vi "ViewWindowCreate.vi"(10 "File":string="FixedHorizonTrans.png", 11 "Solid Horizon Path.PNG":path=path "C:/Users/uksayerr/Documents/My LabView/Content Creation/artificial horizon/FixedHorizonTrans.png") -> (3 "SceneObject out":refnum<vi>)   [LabVIEW 2010]
uses:
  <vilib>/picture/3D Picture Control/NI_3D Picture Control.lvlib
panel:
  # "Generates the Viewing Window with the picture \nat the path specified below"
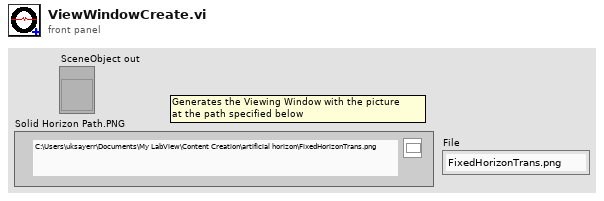
[diagram p1: front panel]
types:
  T1 = enum16{"As a Decal", "With Modulation", "With Blending", "As a replacement"}
  T2 = cluster{"Red":sgl, "Green":sgl, "Blue":sgl, "Alpha":sgl}[]
  T3 = enum16{"Overall", "Per Primitive", "Per Vertex", "Binding Off"}
  T4 = enum16{"Normal Bin", "Opaque Bin", "Transparent Bin"}
  T5 = enum16{"Points", "Lines", "Line Strip", "Line Loop", "Triangles", "Triangle Strip", "Triangle Fan", "Quads", "Quad Strip", "Polygon"}
  T6 = typedef "imagedata.ctl" = cluster{"image type":i32, "image depth":i32, "image":u8[], "mask":u8[], "colors":u32[], "Rectangle":cluster{"left":i16, "top":i16, "right":i16, "bottom":i16}}
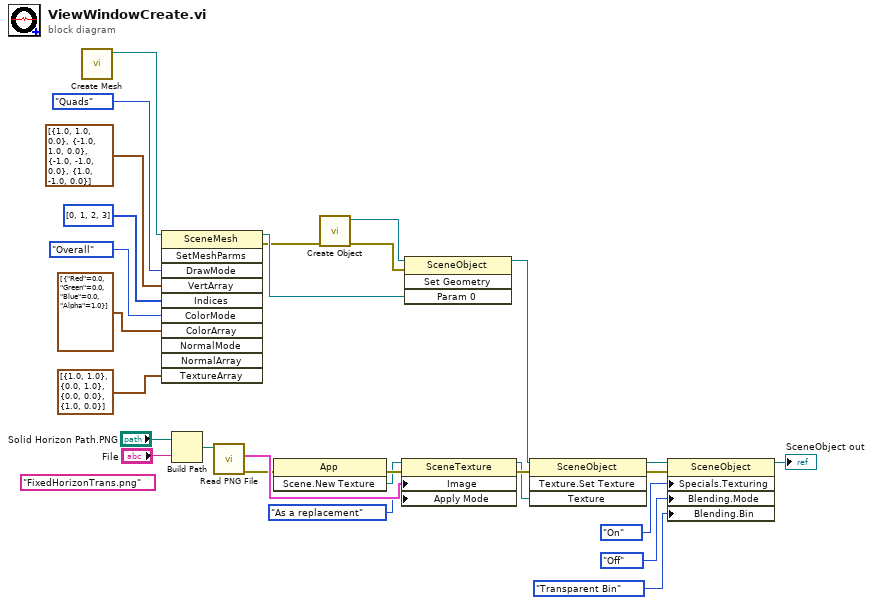
[diagram p0: block diagram]
diagram:
  (unwired) "FixedHorizonTrans.png" ("name or relative path")
  n1 = call <vilib>:"Create Mesh.vi"() -> ("New Mesh Refnum"=w12:refnum<vi>)  [unwired: 10 in, 1 out]
  n2 = invoke class="SceneMesh" method="SetMeshParms"(reference=w12, "DrawMode"=T5."Quads" ("Draw Mode"), "VertArray"=cluster{"X":sgl, "Y":sgl, "Z":sgl}[] [{"X"=1.0, "Y"=1.0, "Z"=0.0}, {"X"=-1.0, "Y"=1.0, "Z"=0.0}, {"X"=-1.0, "Y"=-1.0, "Z"=0.0}, {"X"=1.0, "Y"=-1.0, "Z"=0.0}] ("Vertex Array"), "Indices"=u32[] [0, 1, 2, 3], "ColorMode"=T3."Overall" ("Color Binding Mode"), "ColorArray"=T2 [{"Red"=0.0, "Green"=0.0, "Blue"=0.0, "Alpha"=1.0}] ("Color Array"), "TextureArray"=cluster{"S":sgl, "T":sgl}[] [{"S"=1.0, "T"=1.0}, {"S"=0.0, "T"=1.0}, {"S"=0.0, "T"=0.0}, {"S"=1.0, "T"=0.0}] ("Texture Coordinate Array")) -> (reference out=w19:refnum<vi>, error out=w17:errorcluster)  [unwired: 4 in, 9 out]
  n3 = Build Path(base path="Solid Horizon Path.PNG", name or relative path="File") -> (appended path=w2:path)
  n4 = call <vilib>:"Read PNG File.vi"("path to PNG file"=w2) -> ("error out"=w10:errorcluster, "image data"=w11:T6)  [unwired: 8 in, 1 out]
  n5 = invoke class="App" method="Scene.New Texture"(error in=w10) -> (error out=w8:errorcluster, "Scene.New Texture"=w7:refnum<vi>)  [unwired: 2 in, 1 out]
  n6 = call <vilib>:"Create Object.vi"("error in (no error)"=w17) -> ("error out"=w18:errorcluster, "Scene:New Object"=w5:refnum<vi>)  [unwired: 9 in]
  n7 = property class="SceneTexture"(reference=w7, error in=w8, "Image"=w11, "Apply Mode"=T1."As a replacement") -> (reference out=w20:refnum<vi>, error out=w21:errorcluster)
  n8 = invoke class="SceneObject" method="Set Geometry"(reference=w5, error in=w18, "Param 0"=w19) -> (reference out=w6:refnum<vi>)  [unwired: 1 in, 3 out]
  n9 = invoke class="SceneObject" method="Texture.Set Texture"(reference=w6, error in=w21, "Texture"=w20) -> (reference out=w22:refnum<vi>, error out=w23:errorcluster)  [unwired: 1 in, 2 out]
  n10 = property class="SceneObject"(reference=w22, error in=w23, "Specials.Texturing"=enum16{"Inherit Value", "Off", "On"}."On" ("Specials:Texturing"), "Blending.Mode"=enum16{"Inherit Value", "Off", "On"}."Off" ("Blending:Mode 2"), "Blending.Bin"=T4."Transparent Bin" ("Blending:Bin")) -> (reference out=→"SceneObject out":refnum<vi>)  [unwired: 1 out]
